vi "setListBoxColumnWidths.vi"(1 "table data":string[][](array[string]), 2 "MCListbox Refnum":refnum<vi>) -> ()   [LabVIEW 2020]
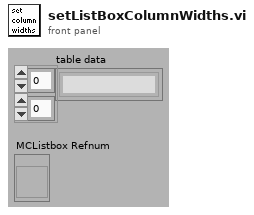
[diagram p1: front panel]
types:
  T1 = enum16{"User-specified Font", "Application Font", "System Font", "Dialog Font"}
  T2 = cluster{"left":i16, "top":i16, "right":i16, "bottom":i16}
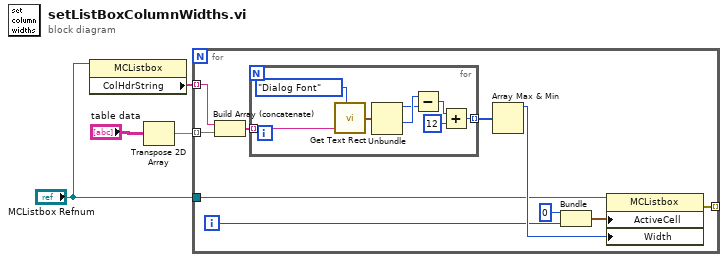
[diagram p0: block diagram]
diagram:
  n1 = property on="Property Node" class="MCListbox"(reference="MCListbox Refnum") -> ("ColHdrString"=w3:string[])  [unwired: 1 in, 2 out]
  n2 = Transpose 2D Array(2D array="table data") -> (transposed array=w1:string[][])
  n3 = for {
    tunnel: w1 -> [w7] mode=indexing
    tunnel: "MCListbox Refnum" -> [w9]
    tunnel: w3 -> [w8] mode=indexing
    tunnel: [w5] -> _ mode=indexing
    i -> [w10]
    n4 = Build Array (concatenate)(w8, w7) -> (w6:string[])
    n5 = for {
      tunnel: [w17] -> w13 mode=indexing
      tunnel: w6 -> [w15] mode=indexing
      n6 = call <vilib>:"Get Text Rect.vi"("desired font(Application)"=T1."Dialog Font", "text"=w15) -> ("rect"=w22:T2)  [unwired: 7 in]
      n7 = Unbundle(w22) -> ("left"=w20:i16, "right"=w21:i16)  [unwired: 2 out]
      n8 = Subtract(x=w21, y=w20) -> (x-y=w19:i16)
      n9 = Add(x=w19, y=i16 12) -> (x+y=w17:i16)
    }
    n10 = Array Max & Min(array=w13) -> (max value=w12:i16)  [unwired: 3 out]
    n11 = Bundle(0, w10) -> (w14:cluster{i32, i32})  [unwired: 1 in]
    n12 = property on="Property Node" class="MCListbox"(reference=w9, "ActiveCell"=w14, "Width"=w12) -> (error out=w5:errorcluster)  [unwired: 1 in, 1 out]
  }
